vi "old tests.vi"   [LabVIEW 2020]
types:
  T1 = typedef "WPI_JoystickDevRef.ctl" = cluster{"Device":T2}
  T2 = typedef "WPI_JoystickDeviceEnum.ctl" = enum16{"USB 0", "USB 1", "USB 2", "USB 3", "USB 4", "USB 5"}
  T3 = typedef "WPI_MotorControlDeviceRef.ctl" = cluster{"DeviceStatus":errorcluster, "Type":T4, "PWM":cluster{"PWM Channel":T5, "DeadBand":T6}, "CAN":cluster{"Device Number":u8, "SetOutput VI Ref":variant, "GetOutput VI Ref":variant, "Enable VI Ref":variant, "Disable VI Ref":variant, "Data":variant}, "Invert":bool, "DIO PWM":cluster{"PWM \"Enable\" Channel":T5, "DIOChannel":T7, "PWM Rate":dbl}}
  T4 = typedef "WPI_MotorControlType.ctl" = enum16{"PWM", "CAN", "DIO PWM"}
  T5 = typedef "FPGA_DIOPWMChannel.ctl" = enum8{"PWM 0", "PWM 1", "PWM 2", "PWM 3", "PWM 4", "PWM 5", "PWM 6", "PWM 7", "PWM 8", "PWM 9", "PWM MXP 0", "PWM MXP 1", "PWM MXP 2", "PWM MXP 3", "PWM MXP 4", "PWM MXP 5", "PWM MXP 6", "PWM MXP 7", "PWM MXP 8", "PWM MXP 9", "Invalid"}
  T6 = typedef "WPI_PWMDeadband.ctl" = cluster{"Name":string, "maxPositivePwm":i32, "minPositivePwm":i32, "centerPwm":i32, "maxNegativePwm":i32, "minNegativePwm":i32, "angularRange":u16}
  T7 = typedef "FPGA_DIOChannel.ctl" = enum8{"DIO 0", "DIO 1", "DIO 2", "DIO 3", "DIO 4", "DIO 5", "DIO 6", "DIO 7", "DIO 8", "DIO 9", "DIO MXP 0", "DIO MXP 1", "DIO MXP 2", "DIO MXP 3", "DIO MXP 4", "DIO MXP 5", "DIO MXP 6", "DIO MXP 7", "DIO MXP 8", "DIO MXP 9", "DIO MXP 10", "DIO MXP 11", "DIO MXP 12", "DIO MXP 13", "DIO MXP 14", "DIO MXP 15", "SPI Port CS1", "SPI Port CS2", "SPI Port CS3", "SPI Port MISO", "SPI Port MOSI", "Invalid"}
  T8 = cluster{"JoystickDevRef":T1, "PhoenixMotorControlDevRef":T3}
  T9 = cluster{"JoystickDevRef":T1, "MotorControlDevRef":T3}
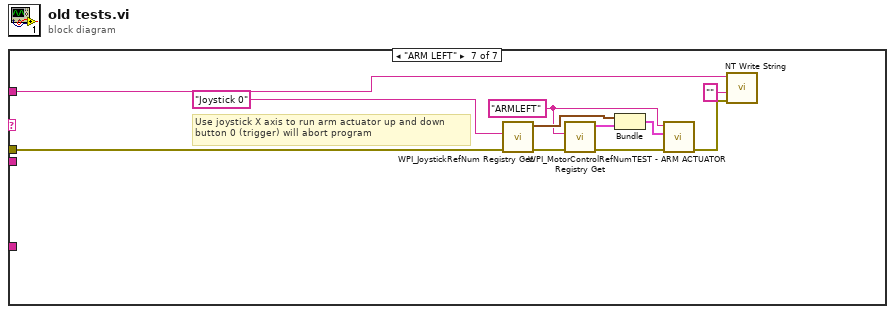
[diagram p0: block diagram]
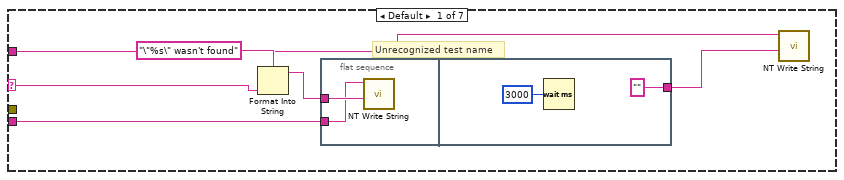
[diagram p2: hidden frame]
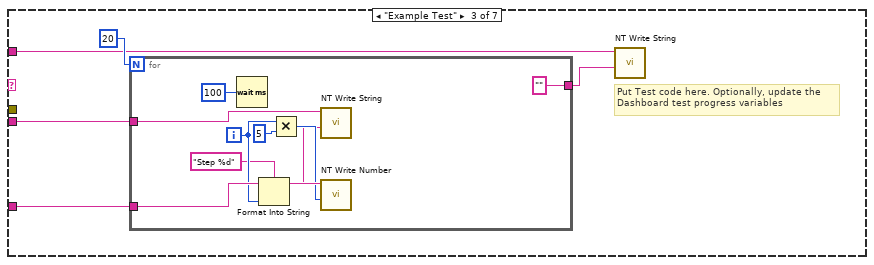
[diagram p4: hidden frame]
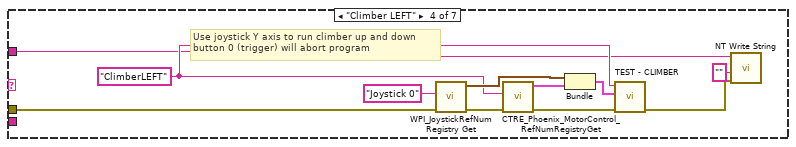
[diagram p5: hidden frame]
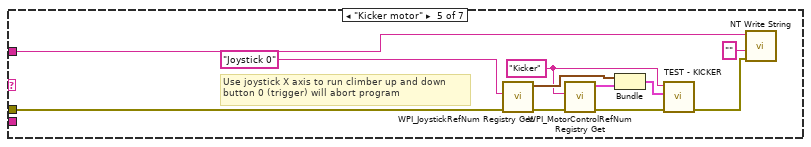
[diagram p6: hidden frame]
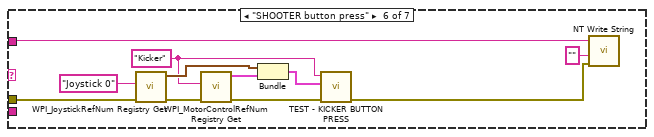
[diagram p7: hidden frame]
diagram:
  n1 = case shown="\"ARM LEFT\"" {
    selector: _ -> [w5 _ _ _ _ _ _]
    tunnel: _ -> [w2 _ w11 w26 w36 w47 w58]
    tunnel: _ -> [w6 _ w14 _ _ _ _]
    tunnel: _ -> [_ _ w15 _ _ _ _]
    tunnel: _ -> [_ _ _ w29 w40 w51 w64]
    frame Default {
      # "Unrecognized test name"
      n2 = Format Into String(format string="\"%s\" wasn't found" ("Name"), w5) -> (resulting string=w4:string)  [unwired: 2 in, 1 out]
      n3 = flat-sequence {
        tunnel: w6 -> [w7]
        tunnel: w4 -> [w8]
        tunnel: ["" ("Name")] -> w1
        frame #0 {
          n4 = call <vilib>:"NT Write String.vi"("String"=w8, "Name"=w7) -> ()  [unwired: 9 in, 1 out]
        }
        frame #1 {
          n5 = Wait (ms)(milliseconds to wait=u32 3000) -> ()  [unwired: 1 out]
        }
      }
      n6 = call <vilib>:"NT Write String.vi"("String"=w1, "Name"=w2) -> ()  [unwired: 9 in, 1 out]
    }
    frame "" {
      # "No test to run"
    }
    frame "Example Test" {
      # "Put Test code here. Optionally, update the\nDashboard test progress variables"
      n7 = for {
        N: 20 -> [_]
        tunnel: w15 -> [w24]
        tunnel: w14 -> [w22]
        tunnel: ["" ("String")] -> w12
        i -> [w19]
        n8 = Wait (ms)(milliseconds to wait=u32 100) -> ()  [unwired: 1 out]
        n9 = Format Into String(format string="Step %d", w19) -> (resulting string=w17:string)  [unwired: 2 in, 1 out]
        n10 = Multiply(x=w19, y=u32 5 ("milliseconds to wait")) -> (x*y=w20:u32)
        n11 = call <vilib>:"NT Write String.vi"("String"=w17, "Name"=w22) -> ()  [unwired: 9 in, 1 out]
        n12 = call <vilib>:"NT Write Number.vi"("Numeric"=w20, "Name"=w24) -> ()  [unwired: 9 in, 1 out]
      }
      n13 = call <vilib>:"NT Write String.vi"("String"=w12, "Name"=w11) -> ()  [unwired: 9 in, 1 out]
    }
    frame "Climber LEFT" {
      w30 = "ClimberLEFT" ("refnum name")
      # "Use joystick Y axis to run climber up and down\nbutton 0 (trigger) will abort program"
      n14 = call <vilib>:"WPI_JoystickRefNum Registry Get.vi"("error in (no error)"=w29, "refnum name"="Joystick 0") -> ("error out"=w31:errorcluster, "JoystickDevRef"=w34:T1)  [unwired: 8 in]
      n15 = call <vilib>:"CTRE_Phoenix_MotorControl_RefNumRegistryGet.vi"("error in (no error)"=w31, "refnum name"=w30) -> ("error out"=w28:errorcluster, "PhoenixMotorControlDevRef"=w33:T3)  [unwired: 8 in]
      n16 = Bundle("JoystickDevRef"=w34, "PhoenixMotorControlDevRef"=w33) -> (w32:T8)  [unwired: 1 in]
      n17 = call "TEST - CLIMBER.vi"("error in (no error)"=w28, "Cluster of JOYSTICK and CLIMBER ref info"=w32, "refnum name"=w30) -> ("error out"=w25:errorcluster)  [unwired: 8 in]
      n18 = call <vilib>:"NT Write String.vi"("error in"=w25, "String"="", "Name"=w26) -> ()  [unwired: 8 in, 1 out]
    }
    frame "Kicker motor" {
      w41 = "Kicker" ("refnum name")
      # "Use joystick X axis to run climber up and down\nbutton 0 (trigger) will abort program"
      n19 = call <vilib>:"WPI_JoystickRefNum Registry Get.vi"("error in (no error)"=w40, "refnum name"="Joystick 0") -> ("error out"=w42:errorcluster, "JoystickDevRef"=w45:T1)  [unwired: 8 in]
      n20 = call <vilib>:"WPI_MotorControlRefNum Registry Get.vi"("error in (no error)"=w42, "refnum name"=w41) -> ("error out"=w39:errorcluster, "MotorControlDevRef"=w44:T3)  [unwired: 8 in]
      n21 = Bundle("JoystickDevRef"=w45, "MotorControlDevRef"=w44) -> (w43:T9)  [unwired: 1 in]
      n22 = call "TEST - KICKER.vi"("error in (no error)"=w39, "Cluster of JOYSTICK and KICKER ref info"=w43, "refnum name"=w41) -> ("error out"=w37:errorcluster)  [unwired: 8 in]
      n23 = call <vilib>:"NT Write String.vi"("error in"=w37, "String"="", "Name"=w36) -> ()  [unwired: 8 in, 1 out]
    }
    frame "SHOOTER button press" {
      w52 = "Kicker" ("refnum name")
      n24 = call <vilib>:"WPI_JoystickRefNum Registry Get.vi"("error in (no error)"=w51, "refnum name"="Joystick 0") -> ("error out"=w53:errorcluster, "JoystickDevRef"=w56:T1)  [unwired: 8 in]
      n25 = call <vilib>:"WPI_MotorControlRefNum Registry Get.vi"("error in (no error)"=w53, "refnum name"=w52) -> ("error out"=w50:errorcluster, "MotorControlDevRef"=w55:T3)  [unwired: 8 in]
      n26 = Bundle("JoystickDevRef"=w56, "MotorControlDevRef"=w55) -> (w54:T9)  [unwired: 1 in]
      n27 = call "TEST - KICKER BUTTON PRESS.vi"("error in (no error)"=w50, "Cluster of JOYSTICK and KICKER ref info"=w54, "refnum name"=w52) -> ("error out"=w49:errorcluster)  [unwired: 8 in]
      n28 = call <vilib>:"NT Write String.vi"("error in"=w49, "String"="", "Name"=w47) -> ()  [unwired: 8 in, 1 out]
    }
    frame "ARM LEFT" {
      w61 = "ARMLEFT" ("refnum name")
      # "Use joystick X axis to run arm actuator up and down\nbutton 0 (trigger) will abort program"
      n29 = call <vilib>:"WPI_JoystickRefNum Registry Get.vi"("error in (no error)"=w64, "refnum name"="Joystick 0") -> ("error out"=w65:errorcluster, "JoystickDevRef"=w67:T1)  [unwired: 8 in]
      n30 = call <vilib>:"WPI_MotorControlRefNum Registry Get.vi"("error in (no error)"=w65, "refnum name"=w61) -> ("error out"=w63:errorcluster, "MotorControlDevRef"=w66:T3)  [unwired: 8 in]
      n31 = Bundle("JoystickDevRef"=w67, "MotorControlDevRef"=w66) -> (w62:T9)  [unwired: 1 in]
      n32 = call "TEST - ARM ACTUATOR.vi"("error in (no error)"=w63, "Cluster of JOYSTICK and ARM ACTUATOR ref info"=w62, "refnum name"=w61) -> ("error out"=w59:errorcluster)  [unwired: 8 in]
      n33 = call <vilib>:"NT Write String.vi"("error in"=w59, "String"="", "Name"=w58) -> ()  [unwired: 8 in, 1 out]
    }
  }
